vi "Time Elapsed Since Last Call.vi"() -> (3 "Time Elapsed Since Last Call [s]":dbl format="%.1p")   [LabVIEW 2020, in "RTAF.lvlib"]
uses:
  RTAF.lvlib
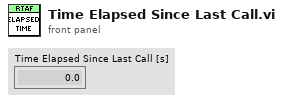
[diagram p1: front panel]
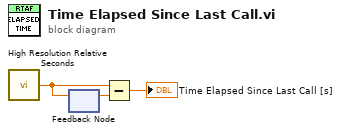
[diagram p0: block diagram]
diagram:
  n1 = call <vilib>:"High Resolution Relative Seconds.vi"() -> ("relative seconds"=w1:dbl)
  n2 = feedback #1() -> (w2:dbl)  [unwired: 1 in]
  n3 = feedback-in #1(w1) -> ()
  n4 = Subtract(x=w1, y=w2) -> (x-y=→"Time Elapsed Since Last Call [s]":dbl)
